vi "Init.vi"(8 "error in (no error)":errorcluster, 10 "Node Reg":refnum<k20>, 11 "Structure in":refnum<class "Structure.lvclass">) -> (0 "error out":errorcluster, 3 "Structure out":refnum<class "Structure.lvclass">)   [LabVIEW 2025, in "Structure.lvclass"]
uses:
  Structure.lvclass
  C:/Users/mrjak/Documents/GitHub/LVGPT/LabVIEW/VIs/Classes/Node/Node.lvclass
  Controls/Subdiagram.ctl
  Controls/Tunnel.ctl
  Controls/Terminal.ctl
  Controls/wire.ctl
  Node.lvclass/Node.ctl
  Node.lvclass
  <vilib>/xml/NI_XML.lvlib
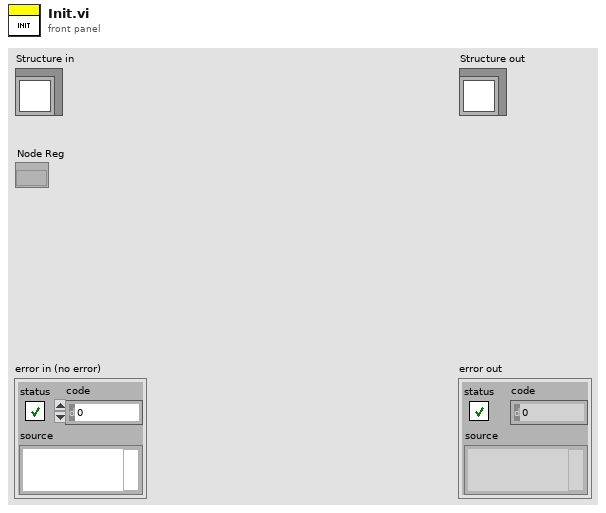
[diagram p1: front panel]
types:
  T1 = typedef "Subdiagram.ctl" = cluster{"diagram":refnum<vi>, "selector":string, "uuid":string}
  T2 = typedef "wire.ctl" = cluster{"id":string, "from":string, "to":string}
  T3 = typedef "Terminal.ctl" = cluster{"id":string, "name":string, "terminal":refnum<vi>}
  T4 = typedef "Tunnel.ctl" = cluster{"OuterUUID":T3, "InnerUUIDs":T3[], "create_wire":T2}
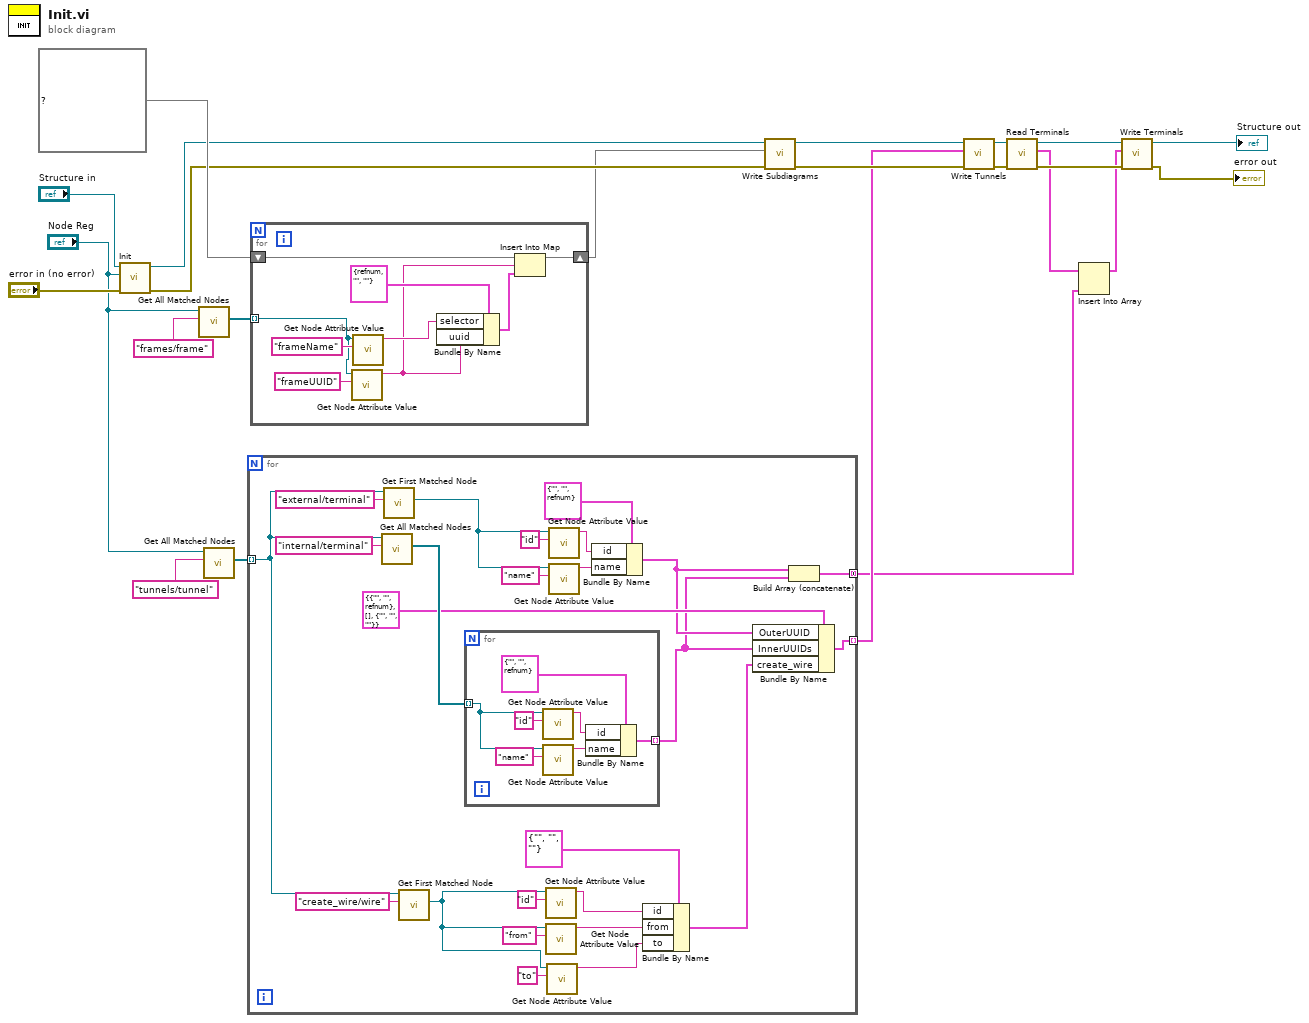
[diagram p0: block diagram]
diagram:
  n1 = call-parent "Init.vi"("error in (no error)"="error in (no error)", "Node Reg"="Node Reg", "Node in"="Structure in") -> ("error out"=w16:errorcluster, "Node out"=w15:refnum<class "Structure.lvclass">)  [unwired: 7 in]
  n2 = call <vilib>:"Get All Matched Nodes.vi"("XPath expression"="frames/frame", "node in"="Node Reg") -> ("node result array"=w20:refnum<k20>[])  [unwired: 7 in, 2 out]
  n3 = call <vilib>:"Get All Matched Nodes.vi"("XPath expression"="tunnels/tunnel", "node in"="Node Reg") -> ("node result array"=w10:refnum<k20>[])  [unwired: 7 in, 2 out]
  n4 = for {
    tunnel: w10 -> [w33] mode=indexing
    tunnel: [w38] -> w4 mode=indexing
    tunnel: [w35] -> w1 mode=concatenating
    n5 = call <vilib>:"Get All Matched Nodes.vi"("XPath expression"="internal/terminal", "node in"=w33) -> ("node result array"=w46:refnum<k20>[])  [unwired: 7 in, 2 out]
    n6 = call <vilib>:"Get First Matched Node.vi"("XPath expression"="external/terminal", "node in"=w33) -> ("node result"=w40:refnum<k20>)  [unwired: 7 in, 2 out]
    n7 = call <vilib>:"Get First Matched Node.vi"("XPath expression"="create_wire/wire", "node in"=w33) -> ("node result"=w24:refnum<k20>)  [unwired: 7 in, 2 out]
    n8 = for {
      tunnel: w46 -> [w55] mode=indexing
      tunnel: [w49] -> w36 mode=indexing
      n9 = call "Get Node Attribute Value.vi"("Attribute Name"="id", "Refnum in"=w55) -> ("Value"=w50:string)  [unwired: 9 in]
      n10 = call "Get Node Attribute Value.vi"("Attribute Name"="name", "Refnum in"=w55) -> ("Value"=w51:string)  [unwired: 9 in]
      n11 = Bundle By Name(cluster=T3 {"id"="", "name"="", "terminal"=refnum} ("Terminal"), "id"=w50, "name"=w51) -> (w49:T3)
    }
    n12 = call "Get Node Attribute Value.vi"("Attribute Name"="id", "Refnum in"=w24) -> ("Value"=w28:string)  [unwired: 9 in]
    n13 = call "Get Node Attribute Value.vi"("Attribute Name"="from", "Refnum in"=w24) -> ("Value"=w27:string)  [unwired: 9 in]
    n14 = call "Get Node Attribute Value.vi"("Attribute Name"="to", "Refnum in"=w24) -> ("Value"=w26:string)  [unwired: 9 in]
    n15 = call "Get Node Attribute Value.vi"("Attribute Name"="id", "Refnum in"=w40) -> ("Value"=w41:string)  [unwired: 9 in]
    n16 = call "Get Node Attribute Value.vi"("Attribute Name"="name", "Refnum in"=w40) -> ("Value"=w42:string)  [unwired: 9 in]
    n17 = Bundle By Name(cluster=T3 {"id"="", "name"="", "terminal"=refnum} ("Terminal"), "id"=w41, "name"=w42) -> (w37:T3)
    n18 = Bundle By Name(cluster=T2 {"id"="", "from"="", "to"=""} ("Wire"), "id"=w28, "from"=w27, "to"=w26) -> (w25:T2)
    n19 = Bundle By Name(cluster=T4 {"OuterUUID"={"id"="", "name"="", "terminal"=refnum}, "InnerUUIDs"=[], "create_wire"={"id"="", "from"="", "to"=""}} ("Tunnel"), "OuterUUID"=w37, "InnerUUIDs"=w36, "create_wire"=w25) -> (w38:T4)
    n20 = Build Array (concatenate)(w37, w36) -> (w35:T3[])
  }
  n21 = for {
    tunnel: w20 -> [w62] mode=indexing
    shift-right: [w60] -> w13
    shift-left: map{string, T1} {} ("Subdiagrams") -> [w61]
    n22 = call "Get Node Attribute Value.vi"("Attribute Name"="frameUUID", "Refnum in"=w62) -> ("Value"=w56:string)  [unwired: 9 in]
    n23 = call "Get Node Attribute Value.vi"("Attribute Name"="frameName", "Refnum in"=w62) -> ("Value"=w57:string)  [unwired: 9 in]
    n24 = Bundle By Name(cluster=T1 {"diagram"=refnum, "selector"="", "uuid"=""} ("value"), "selector"=w57, "uuid"=w56) -> (w58:T1)
    n25 = Insert Into Map(map in=w61, key=w56, value=w58) -> (map out=w60:map{string, T1})  [unwired: 2 out]
  }
  n26 = call-dynamic "Write Subdiagrams.vi"("error in (no error)"=w16, "Subdiagrams"=w13, "Structure in"=w15) -> ("error out"=w18:errorcluster, "Structure out"=w19:refnum<class "Structure.lvclass">)  [unwired: 7 in]
  n27 = call-dynamic "Write Tunnels.vi"("error in (no error)"=w18, "Tunnels"=w4, "Structure in"=w19) -> ("error out"=w7:errorcluster, "Structure out"=w14:refnum<class "Structure.lvclass">)  [unwired: 7 in]
  n28 = call "Read Terminals.vi"("error in (no error)"=w7, "Node in"=w14) -> ("error out"=w6:errorcluster, "Terminals"=w3:T3[], "Node out"=w8:refnum<class "Structure.lvclass">)  [unwired: 7 in]
  n29 = Insert Into Array(array=w3, new element=w1) -> (w2:T3[])  [unwired: 1 in]
  n30 = call "Write Terminals.vi"("error in (no error)"=w6, "Terminals"=w2, "Node in"=w8) -> ("error out"=→"error out":errorcluster, "Node out"=→"Structure out":refnum<class "Structure.lvclass">)  [unwired: 7 in]
